vi "Tosca-Process Adaptive Tracking Response.vi"(0 "Track in":T1, 5 "Result":T3, 9 "Track":T4) -> (4 "Track out":T1, 6 "change":bool, 10 "catch is tracked":bool, 13 "reversal":bool, 14 "Finished":bool)   [LabVIEW 2020]
uses:
  Typedefs/Tosca-Adaptive Track.ctl
  Typedefs/Tosca-Simple Variable.ctl
  Adaptation VIs/Tosca-Adapt Threshold Metric.ctl
  Typedefs/Tosca-Trial Result Enum.ctl
  Typedefs/Tosca-Adaptation Track State.ctl
  Typedefs/Tosca-Adaptation History Element.ctl
  <vilib>/Analysis/baseanly.llb/Mean (DBL).vi
  <vilib>/Analysis/NI_AALBase.lvlib
  <vilib>/gmath/NI_Gmath.lvlib
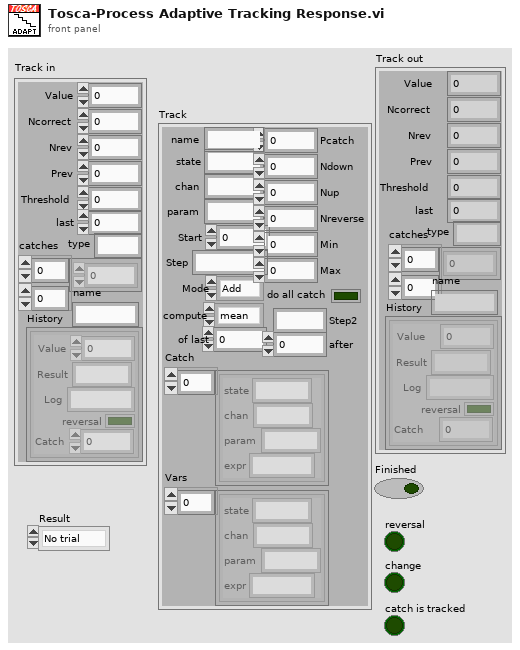
[diagram p1: front panel]
types:
  T1 = typedef "Tosca-Adaptation Track State.ctl" = cluster{"Value":dbl, "Ncorrect":i32, "Nrev":i32, "Prev":dbl, "History":T2[], "Threshold":dbl, "last":i32, "type":string, "catches":dbl[][], "name":string}
  T2 = typedef "Tosca-Adaptation History Element.ctl" = cluster{"Value":dbl, "Result":string, "Log":string, "reversal":bool, "Catch":dbl}
  T3 = typedef "Tosca-Trial Result Enum.ctl" = enum16{"No trial", "Go", "No go", "Error", "Abort"}
  T4 = typedef "Tosca-Adaptive Track.ctl" = cluster{"state":string, "chan":string, "param":string, "Start":dbl, "Step":string, "Mode":enum16{"Add", "Multiply"}, "Pcatch":dbl, "Ndown":i32, "Nup":i32, "Nreverse":i32, "Min":dbl, "Max":dbl, "Catch":T5[], "do all catch":bool, "name":string, "Vars":T5[], "compute":T6, "of last":i32, "Step2":string, "after":i32}
  T5 = typedef "Tosca-Simple Variable.ctl" = cluster{"state":string, "chan":string, "param":string, "expr":string}
  T6 = typedef "Tosca-Adapt Threshold Metric.ctl" = enum16{"mean", "median"}
  T7 = cluster{"Value":dbl, string, string, bool, "f":dbl}
  T8 = cluster{"Value":dbl, string, string, bool, "Value 2":dbl}
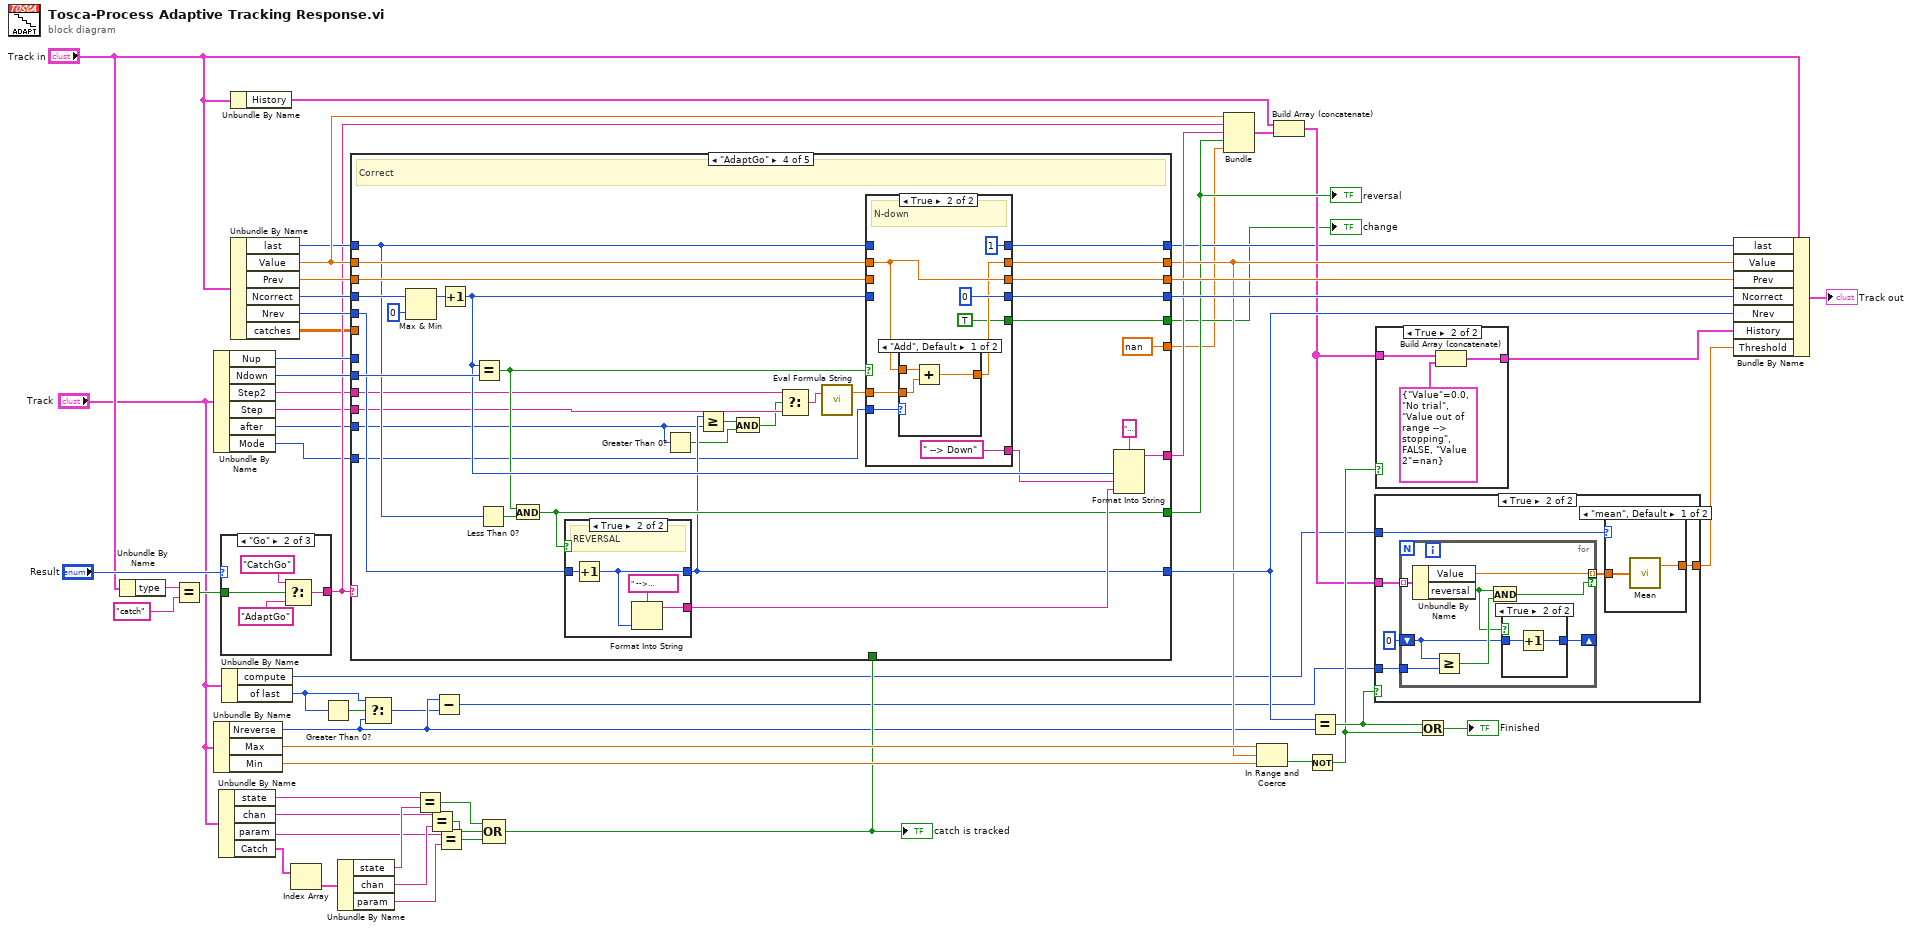
[diagram p0: block diagram]
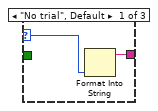
[diagram p2: hidden frame]
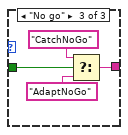
[diagram p3: hidden frame]
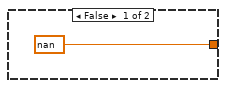
[diagram p5: hidden frame]
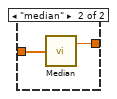
[diagram p6: hidden frame]
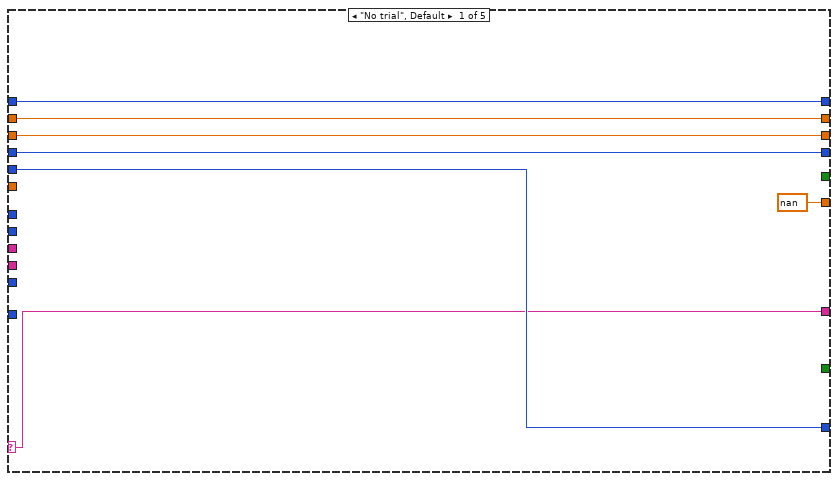
[diagram p8: hidden frame]
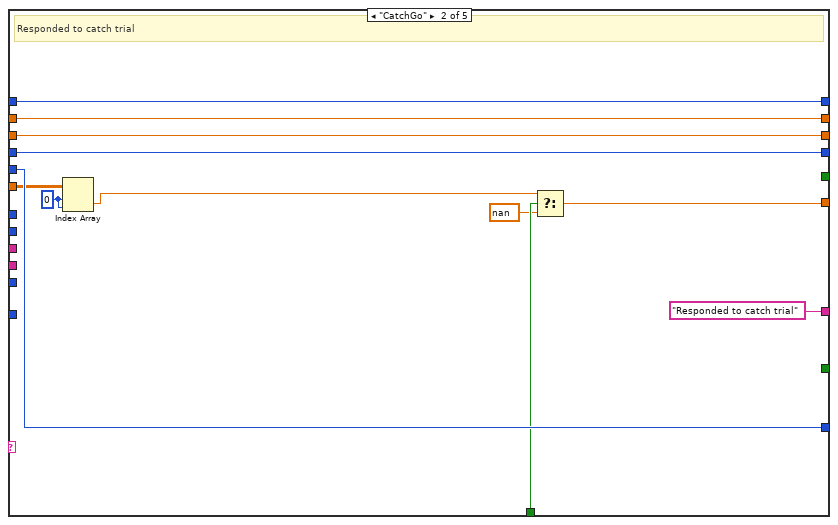
[diagram p9: hidden frame]
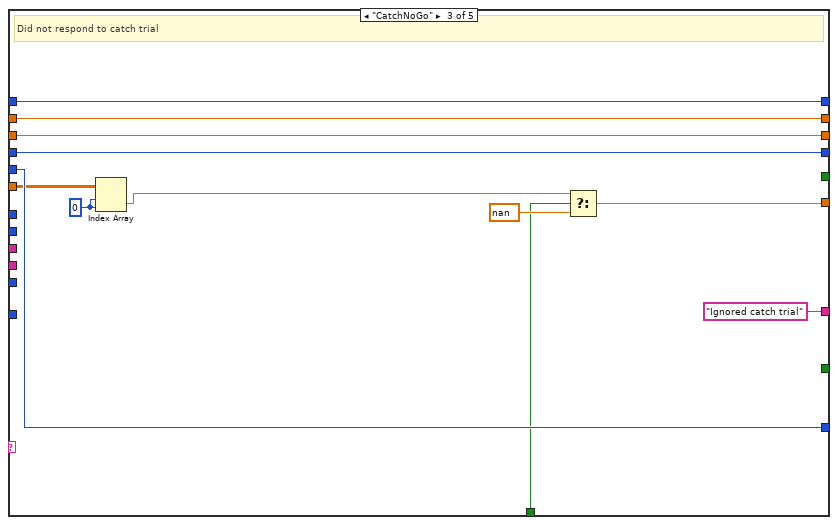
[diagram p10: hidden frame]
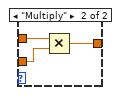
[diagram p12: hidden frame]
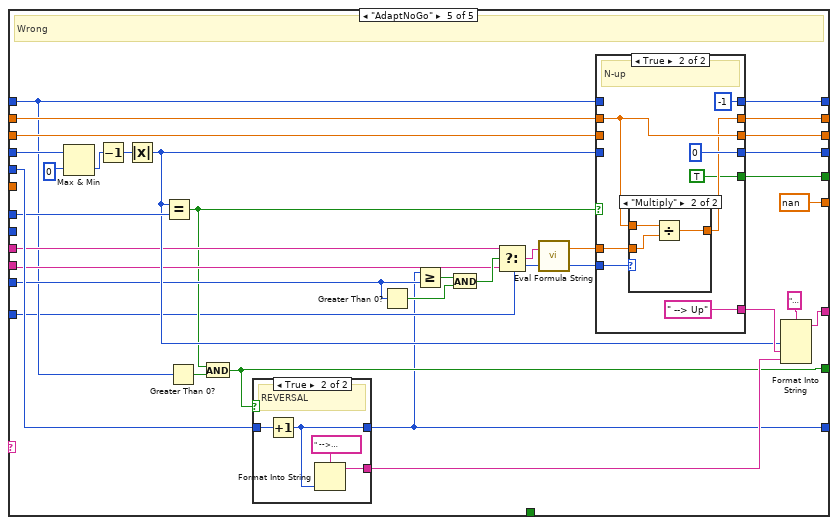
[diagram p14: hidden frame]
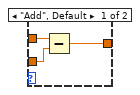
[diagram p16: hidden frame]
diagram:
  n1 = Unbundle By Name("Track in") -> ("type"=w29:string)
  n2 = Equal?(x=w29, y="catch") -> (x = y?=w28:bool)
  n3 = Unbundle By Name("Track") -> ("Nup"=w51:i32, "Ndown"=w53:i32, "Step2"=w4:string, "Step"=w3:string, "after"=w2:i32, "Mode"=w1:enum16{"Add", "Multiply"})
  n4 = Unbundle By Name("Track") -> ("Nreverse"=w7:i32, "Max"=w46:dbl, "Min"=w45:dbl)
  n5 = Unbundle By Name("Track") -> ("state"=w23:string, "chan"=w21:string, "param"=w19:string, "Catch"=w25:T5[])
  n6 = case shown="\"Go\"" "Result" {
    selector: "Result" -> [w59 _ _]
    tunnel: w28 -> [_ w64 w68]
    tunnel: [w60 w61 w65] -> w32
    frame "No trial", Default {
      n7 = Format Into String(w59) -> (resulting string=w60:string)  [unwired: 3 in, 1 out]
    }
    frame "Go" {
      n8 = Select(t="CatchGo", s=w64, f="AdaptGo") -> (s? t:f=w61:string)
    }
    frame "No go" {
      n9 = Select(t="CatchNoGo", s=w68, f="AdaptNoGo") -> (s? t:f=w65:string)
    }
  }
  n10 = Unbundle By Name("Track") -> ("compute"=w10:T6, "of last"=w8:i32)
  n11 = Unbundle By Name("Track in") -> ("History"=w49:T2[])
  n12 = Unbundle By Name("Track in") -> ("last"=w35:i32, "Value"=w50:dbl, "Prev"=w57:dbl, "Ncorrect"=w56:i32, "Nrev"=w55:i32, "catches"=w14:dbl[][])
  n13 = Index Array(array=w25) -> (element=w24:T5)  [unwired: 1 in]
  n14 = Greater Than 0?(x=w8) -> (x > 0?=w9:bool)
  n15 = Unbundle By Name(w24) -> ("state"=w22:string, "chan"=w20:string, "param"=w18:string)
  n16 = Select(t=w8, s=w9, f=w7) -> (s? t:f=w6:i32)
  n17 = Equal?(x=w23, y=w22) -> (x = y?=w17:bool)
  n18 = Equal?(x=w21, y=w20) -> (x = y?=w16:bool)
  n19 = Subtract(x=w7, y=w6) -> (x-y=w5:i32)
  n20 = Equal?(x=w19, y=w18) -> (x = y?=w15:bool)
  n21 = Compound Arithmetic op=OR(w17, w16, w15) -> (w13:bool)
  "catch is tracked" <- w13
  n22 = case shown="\"AdaptGo\"" w32 {
    selector: w32 -> [w70 _ _ _ _]
    tunnel: w50 -> [w75 w83 w99 w122 w180]
    tunnel: [w75 w83 w99 w123 w181] -> w44
    tunnel: [w74 w87 w98 w124 w182] -> w58
    tunnel: w57 -> [w74 w87 w98 w125 w183]
    tunnel: w56 -> [w73 w82 w97 w128 w186]
    tunnel: w55 -> [w72 w86 w96 w127 w185]
    tunnel: [w73 w82 w97 w126 w184] -> w54
    tunnel: [w72 w86 w96 w105 w155] -> w52
    tunnel: w53 -> [_ _ _ w131 _]
    tunnel: w51 -> [_ _ _ _ w179]
    tunnel: [w70 "Responded to catch trial" "Ignored catch trial" w117 w173] -> w47
    tunnel: [_ _ _ w110 w157] -> w41
    tunnel: w35 -> [w71 w84 w94 w113 w158]
    tunnel: [w71 w84 w94 w114 w169] -> w34
    tunnel: [_ _ _ w116 w171] -> w26
    tunnel: w14 -> [_ w81 w91 _ _]
    tunnel: w13 -> [_ w79 w88 _ _]
    tunnel: [nan ("f") w76 w89 nan ("f") nan ("f")] -> w12
    tunnel: w4 -> [_ _ _ w108 w163]
    tunnel: w3 -> [_ _ _ w106 w162]
    tunnel: w2 -> [_ _ _ w103 w161]
    tunnel: w1 -> [_ _ _ w100 w156]
    frame "No trial", Default {
    }
    frame "CatchGo" {
      w80 = 0 ("index (row)")
      # "Responded to catch trial"
      n23 = Index Array(array=w81, index (row)=w80, index (col)=w80) -> (element=w78:dbl)
      n24 = Select(t=w78, s=w79, f=nan) -> (s? t:f=w76:dbl)
    }
    frame "CatchNoGo" {
      w90 = 0 ("index (row)")
      # "Did not respond to catch trial"
      n25 = Index Array(array=w91, index (row)=w90, index (col)=w90) -> (element=w93:dbl)
      n26 = Select(t=w93, s=w88, f=nan) -> (s? t:f=w89:dbl)
    }
    frame "AdaptGo" {
      # "Correct"
      n27 = Max & Min(x=w128, y=0) -> (max(x,y)=w129:i32)  [unwired: 1 out]
      n28 = Increment(x=w129) -> (x+1=w120:i32)
      n29 = Equal?(x=w120, y=w131) -> (x = y?=w111:bool)
      n30 = Less Than 0?(x=w113) -> (x < 0?=w112:bool)
      n31 = And(x=w111, y=w112) -> (x .and. y?=w110:bool)
      n32 = case shown="True" w110 {
        tunnel: w127 -> [w150 w154]
        tunnel: [w150 w152] -> w105
        tunnel: [_ w151] -> w119
        frame False {
        }
        frame True {
          # "REVERSAL"
          n33 = Increment(x=w154) -> (x+1=w152:i32)
          n34 = Format Into String(format string=" --> REVERSAL #%d", w152) -> (resulting string=w151:string)  [unwired: 2 in, 1 out]
        }
      }
      n35 = Greater Than 0?(x=w103) -> (x > 0?=w102:bool)
      n36 = Greater Or Equal?(x=w105, y=w103) -> (x >= y?=w104:bool)
      n37 = And(x=w104, y=w102) -> (x .and. y?=w101:bool)
      n38 = Select(t=w108, s=w101, f=w106) -> (s? t:f=w107:string)
      n39 = call <vilib>:"Eval Formula String.vi"("formula"=w107) -> ("y value"=w109:dbl)  [unwired: 1 in, 1 out]
      n40 = case shown="True" w111 {
        tunnel: w120 -> [w135 _]
        tunnel: [w135 0] -> w126
        tunnel: w125 -> [w134 _]
        tunnel: [w134 w140] -> w124
        tunnel: [w133 w139] -> w123
        tunnel: w122 -> [w133 w140]
        tunnel: w109 -> [_ w141]
        tunnel: w100 -> [_ w142]
        tunnel: [_ " --> Down"] -> w118
        tunnel: w113 -> [w132 _]
        tunnel: [w132 1] -> w114
        tunnel: [_ TRUE] -> w116
        frame False {
        }
        frame True {
          # "N-down"
          n41 = case shown="\"Add\", Default" w142 {
            tunnel: w141 -> [w145 w148]
            tunnel: w140 -> [w146 w149]
            tunnel: [w144 w147] -> w139
            frame "Add", Default {
              n42 = Add(x=w146, y=w145) -> (x+y=w144:dbl)
            }
            frame "Multiply" {
              n43 = Multiply(x=w149, y=w148) -> (x*y=w147:dbl)
            }
          }
        }
      }
      n44 = Format Into String(format string="%d correct%s%s", w120, w118, w119) -> (resulting string=w117:string)  [unwired: 2 in, 1 out]
    }
    frame "AdaptNoGo" {
      # "Wrong"
      n45 = Max & Min(x=w186, y=0) -> (min(x,y)=w178:i32)  [unwired: 1 out]
      n46 = Decrement(x=w178) -> (x-1=w176:i32)
      n47 = Absolute Value(x=w176) -> (abs(x)=w172:i32)
      n48 = Equal?(x=w172, y=w179) -> (x = y?=w159:bool)
      n49 = Greater Than 0?(x=w158) -> (x > 0?=w160:bool)
      n50 = And(x=w159, y=w160) -> (x .and. y?=w157:bool)
      n51 = case shown="True" w157 {
        tunnel: w185 -> [w206 w210]
        tunnel: [w206 w208] -> w155
        tunnel: [_ w207] -> w174
        frame False {
        }
        frame True {
          # "REVERSAL"
          n52 = Increment(x=w210) -> (x+1=w208:i32)
          n53 = Format Into String(format string=" --> REVERSAL #%d", w208) -> (resulting string=w207:string)  [unwired: 2 in, 1 out]
        }
      }
      n54 = Greater Than 0?(x=w161) -> (x > 0?=w167:bool)
      n55 = Greater Or Equal?(x=w155, y=w161) -> (x >= y?=w168:bool)
      n56 = And(x=w168, y=w167) -> (x .and. y?=w166:bool)
      n57 = Select(t=w163, s=w166, f=w162) -> (s? t:f=w164:string)
      n58 = call <vilib>:"Eval Formula String.vi"("formula"=w164) -> ("y value"=w165:dbl)  [unwired: 1 in, 1 out]
      n59 = case shown="True" w159 {
        tunnel: w172 -> [w191 _]
        tunnel: [w191 0] -> w184
        tunnel: w183 -> [w190 _]
        tunnel: [w190 w196] -> w182
        tunnel: [w189 w195] -> w181
        tunnel: w180 -> [w189 w196]
        tunnel: w165 -> [_ w197]
        tunnel: w156 -> [_ w198]
        tunnel: [_ " --> Up"] -> w175
        tunnel: w158 -> [w188 _]
        tunnel: [w188 -1] -> w169
        tunnel: [_ TRUE] -> w171
        frame False {
        }
        frame True {
          # "N-up"
          n60 = case shown="\"Multiply\"" w198 {
            tunnel: w197 -> [w201 w204]
            tunnel: w196 -> [w202 w205]
            tunnel: [w200 w203] -> w195
            frame "Add", Default {
              n61 = Subtract(x=w202, y=w201) -> (x-y=w200:dbl)
            }
            frame "Multiply" {
              n62 = Divide(x=w205, y=w204) -> (x/y=w203:dbl)
            }
          }
        }
      }
      n63 = Format Into String(format string="%d wrong%s%s", w172, w175, w174) -> (resulting string=w173:string)  [unwired: 2 in, 1 out]
    }
  }
  "reversal" <- w41
  "change" <- w26
  n64 = Bundle("Value"=w50, w32, w47, w41, "f"=w12) -> (w48:T7)  [unwired: 1 in]
  n65 = In Range and Coerce(upper limit=w46, x=w44, lower limit=w45) -> (In Range?=w42:bool)  [unwired: 1 out]
  n66 = Build Array (concatenate)(w49, w48) -> (w37:T2[])
  n67 = Not(x=w42) -> (.not. x?=w39:bool)
  n68 = Equal?(x=w52, y=w7) -> (x = y?=w40:bool)
  n69 = case shown="True" w40 {
    tunnel: w37 -> [_ w217]
    tunnel: [nan ("median") w215] -> w36
    tunnel: w10 -> [_ w213]
    tunnel: w5 -> [_ w214]
    frame False {
    }
    frame True {
      n70 = for {
        tunnel: w217 -> [w229] mode=indexing
        tunnel: [w228] -> w216 mode=indexing if=w226
        tunnel: w214 -> [w227]
        shift-right: [w223] -> _
        shift-left: 0 -> [w224]
        n71 = Unbundle By Name(w229) -> ("Value"=w228:dbl, "reversal"=w222:bool)
        n72 = Greater Or Equal?(x=w224, y=w227) -> (x >= y?=w225:bool)
        n73 = And(x=w222, y=w225) -> (x .and. y?=w226:bool)
        n74 = case shown="True" w222 {
          tunnel: w224 -> [w230 w232]
          tunnel: [w230 w231] -> w223
          frame False {
          }
          frame True {
            n75 = Increment(x=w232) -> (x+1=w231:i32)
          }
        }
      }
      n76 = case shown="\"mean\", Default" w213 {
        tunnel: w216 -> [w219 w221]
        tunnel: [w218 w220] -> w215
        frame "mean", Default {
          n77 = call-poly <vilib>:"Mean.vi"("X"=w219) -> ("mean"=w218:dbl)  [unwired: 1 out]
        }
        frame "median" {
          n78 = call <vilib>:"Median.vi"("X"=w221) -> ("median"=w220:dbl)  [unwired: 1 out]
        }
      }
    }
  }
  n79 = case shown="True" w39 {
    tunnel: w37 -> [w233 w236]
    tunnel: [w233 w235] -> w38
    frame False {
    }
    frame True {
      n80 = Build Array (concatenate)(w236, T8 {"Value"=0.0, "No trial", "Value out of range --> stopping", FALSE, "Value 2"=nan} ("output cluster")) -> (w235:T2[])
    }
  }
  n81 = Or(x=w40, y=w39) -> (x .or. y?=→"Finished":bool)
  n82 = Bundle By Name(cluster="Track in", "last"=w34, "Value"=w44, "Prev"=w58, "Ncorrect"=w54, "Nrev"=w52, "History"=w38, "Threshold"=w36) -> (→"Track out":T1)
